vi "Create VI Snippets.vi"(6 "Skip":cluster{"Functions":i32[], "Controls":i32[]}={"Functions"=[2371, 2060], "Controls"=[3503, 21820]}, 8 "error in (no error)":errorcluster, 9 "Scripting Ring":refnum<vi>, 10 "Type":enum8{"Functions", "Controls"}(ring), 11 "OutputDir":path) -> (0 "error out":errorcluster, 3 "IDs":i32[](array[numeric]))   [LabVIEW 2018, in "Export-Built-ins.lvlib"]
uses:
  Export-Built-ins.lvlib
  <vilib>/Utility/miscctls.llb/LVPointTypeDef.ctl
panel:
  out "Name":string
  out "Current":i32
  out "Last Snippet (.png)":path
  out "Image":picture
  out "Info":string
  out "Last":i32
  out "Remaining":i32
  out "LabVIEW 2018 Scripting Ring":i32(ring)=2125 items=[".NET Container"=2125, ".NET Refnum"=3441, "2D Picture"=3508, "3D Picture"=23776, "Absolute Value"=1054, "Access Rights"=1412, "ActiveX Container"=2072, "Add"=1050, "Add (with error terminals)"=3915, "Add Array Elements"=1903, "Agitator"=3831, "AllSpoll"=1960, "Always Copy"=2400, "And"=1061, "And Array Elements"=1911, "Append True/False String"=1511, "Application Refnum"=3412, "Array (block diagram constant)"=2070, "Array (classic)"=3300, "Array (modern)"=21608, "Array Interface Control"=23777, "Array Max & Min"=1907, "Array of Strings to Path"=1422, "Array Size"=1809, "Array Subset"=2044, "Array To Cluster"=1168, "Array To Spreadsheet String"=1540, "ArrayMemInfo"=2412, "Assert Structural Type Match"=2416, "Atmospheric Tank (classic)"=3070, "Atmospheric Tank (modern)"=21751, "Automation Close"=8001, "Automation Open"=8000, "Automation Refnum"=3410, "Avogadro Constant (1/mol)"=23520, "Base 10 Logarithm Of e"=23512, "Bin #1"=3073, "Bin #2"=21755, "Bitpack to Array"=3135, "Bluetooth Close Connection"=9148, "Bluetooth Create Listener"=9151, "Bluetooth Discover"=9152, "Bluetooth Network Connection Refnum"=3468, "Bluetooth Open Connection"=9153, "Bluetooth Read"=9149, "Bluetooth Wait On Listener"=9147, "Bluetooth Write"=9150, "Boolean Array To Number"=1815, "Boolean To (0,1)"=1167, "Build Array"=2041, "Build Cluster Array"=2047, "Build Matrix"=8500, "Build Path"=1419, "Build Waveform"=2066, "Bundle"=2049, "Bundle By Name"=2057, "Byte Array To String"=1609, "Byte Stream File Refnum"=3408, "Call By Reference"=3901, "Call Chain"=1999, "Call Library Function Node"=2062, "Call Parent Method"=2354, "CAN Channel (block diagram constant)"=2124, "CAN Channel (classic)"=3340, "CAN Channel (modern)"=21817, "CAN Channel (system)"=21966, "CAN Interface (block diagram constant)"=2123, "CAN Interface (classic)"=3339, "CAN Interface (modern)"=21815, "CAN Interface (system)"=21964, "CAN Task (block diagram constant)"=3471, "CAN Task (classic)"=3470, "CAN Task (modern)"=21789, "CAN Task (system)"=21963, "Cancel Button (modern)"=21739, "Cancel Button (system)"=3131, "Cancel Notification"=9107, "Carriage Return Constant"=23500, "Case Structure"=2001, "Cast Unit Bases"=1079, "Check Valve"=3833, "Checkbox (classic)"=3117, "CheckBox (modern)"=21924, "Checkbox (system)"=3132, "Class Specifier Constant"=2094, "Classic Color Box"=3013, "Classic Color Ramp"=3022, "Classic Horizontal Slide Switch"=3114, "Classic Vertical Slide"=3004, "Clear Fixed-Point Overflow Status"=5562, "Close File"=8052, "Close File (deprecated)"=1405, "Close Python Session"=24207, "Close Reference"=8011, "Close Variable Connection"=23783, "Closure Structure"=2372, "Cluster (classic)"=3400, "Cluster (modern)"=21607, "Cluster Constant"=2071, "Cluster To Array"=1169, "Code Interface Node"=2050, "Coerce To Type"=2402, "Color Box Constant"=2120, "Color Box Thin Border"=2905, "Colored Rectangle (broken?)"=3625, "Combo Box (classic)"=3304, "Combo Box (modern)"=21604, "Combo Box (system)"=21917, "Combo Box Constant"=2088, "Complex Conjugate"=1048, "Complex To Polar"=1045, "Complex To Re/Im"=1044, "Compound Arithmetic"=2200, "Compressor"=3832, "Concatenate Strings"=2040, "Conditional Disable Structure"=2064, "Constructor Node"=3904, "Control & Simulation Loop"=2099, "Control Help Window"=1353, "Control Online Help"=1355, "Control Refnum"=3419, "Convert Unit"=2059, "Conveyer"=3827, "Copy"=8053, "Copy (deprecated)"=1416, "Cosecant"=1204, "Cosine"=1201, "Cotangent"=1205, "CPU Information"=24130, "Create Folder"=8055, "Create Network Stream Endpoint"=23793, "Create Network Stream Reader Endpoint"=23811, "Create Network Stream Writer Endpoint"=23810, "Create Stream"=23796, "Create Unique Network Stream Endpoint"=23795, "Create Unique Network Stream Reader Endpoint"=23807, "Create Unique Network Stream Writer Endpoint"=23806, "Create User Event"=2073, "Current Processor ID"=24131, "Current VI's Menubar"=9000, "Current VI's Path"=1426, "DAQmx Analog Trigger Source (block diagram constant)"=2119, "DAQmx Analog Trigger Source (classic)"=3336, "DAQmx Analog Trigger Source (modern)"=21774, "DAQmx Analog Trigger Source (system)"=21951, "DAQmx Device Name (block diagram constant)"=2093, "DAQmx Device Name (classic)"=3318, "DAQmx Device Name (modern)"=21773, "DAQmx Device Name (system)"=21950, "DAQmx Global Channel (block diagram constant)"=3430, "DAQmx Global Channel (classic)"=3443, "DAQmx Global Channel (modern)"=21770, "DAQmx Global Channel (system)"=21957, "DAQmx Physical Channel (block diagram constant)"=2118, "DAQmx Physical Channel (classic)"=3335, "DAQmx Physical Channel (modern)"=21777, "DAQmx Physical Channel (system)"=21954, "DAQmx Scale Name (block diagram constant)"=2116, "DAQmx Scale Name (classic)"=3317, "DAQmx Scale Name (modern)"=21775, "DAQmx Scale Name (system)"=21952, "DAQmx Switch (block diagram constant)"=2121, "DAQmx Switch (classic)"=3337, "DAQmx Switch (modern)"=21776, "DAQmx Switch (system)"=21953, "DAQmx Task Name (block diagram constant)"=3434, "DAQmx Task Name (classic)"=3442, "DAQmx Task Name (modern)"=21778, "DAQmx Task Name (system)"=21959, "DAQmx Terminal (block diagram constant)"=2117, "DAQmx Terminal (classic)"=3319, "DAQmx Terminal (modern)"=21781, "DAQmx Terminal (system)"=21955, "Data Cache Size"=24132, "Data Log File Refnum"=3402, "Data Value Reference"=3476, "Data Value Reference Constant"=24134, "DataSocket Close"=1085, "DataSocket Open"=1084, "DataSocket Read"=1086, "DataSocket Refnum"=3417, "DataSocket Write"=1087, "Date/Time To Seconds"=1308, "Decimal Digit?"=1119, "Decimal String To Number"=1184, "Decimate 1D Array"=2046, "DecomposeLockDataValRef"=2406, "DecomposeVariant"=2404, "Decrement"=1058, "Default Directory"=1427, "Delete"=8056, "Delete (deprecated)"=1417, "Delete Data Value Reference"=2409, "Delete From Array"=3912, "Delete Menu Items"=9004, "Delete Variant Attribute"=8206, "Delete Waveform Attribute"=8209, "Deny Access"=8057, "Dequeue Element"=9113, "Destroy Stream Endpoint"=23794, "Destroy User Event"=2075, "DevClear"=1961, "DevClearList"=1962, "Device Control/Status"=1433, "Device Refnum"=3405, "Diagram Disable Structure"=2054, "Dial (classic)"=3050, "Dial (modern)"=21732, "Digital Data (classic)"=3210, "Digital Data (modern)"=21216, "Digital Waveform Graph (classic)"=3511, "Digital Waveform Graph (modern)"=21718, "Direct Variable Read"=23785, "Direct Variable Write"=23788, "Divide"=1053, "Divide (with error terminals)"=3918, "Dlg Horiz Scrollbar"=21905, "Dlg Mac Group Box"=32514, "Dlg Numeric #1"=2100, "Dlg Numeric #2"=3006, "Dlg String"=2110, "Dlg Vert Scrollbar"=21906, "Down Arrow"=3824, "Down Bow Valve (flat)"=3707, "Down Bow Valve (outline)"=3807, "Down Bow Valve (shaded)"=21767, "Down Rect Valve (flat)"=3706, "Down Rect Valve (outline)"=3806, "Down Rect Valve (shaded)"=21766, "Down Tee (flat)"=3818, "Down Tee (shaded)"=3718, "Dynamic FPGA Interface Cast"=5690, "Eased Corner Rectangle"=32513, "Elementary Charge (C)"=23517, "Empty Array?"=23063, "Empty Path Constant"=23523, "Empty String Constant"=23503, "Empty String/Path?"=1112, "Enable Menu Tracking"=9002, "EnableLocal"=1963, "EnableRemote"=1964, "End of Line Constant"=23525, "Enqueue Element"=9111, "Enqueue Element At Opposite End"=9129, "Enum (classic)"=3023, "Enum (modern)"=21605, "Enum (system)"=3062, "Enum Constant"=2090, "EOF"=1410, "Equal To 0?"=1113, "Equal?"=1102, "Error Ring Constant"=2039, "Event Callback Refnum"=3435, "Event Data Node"=2102, "Event Structure"=2052, "Exchanger"=3828, "Exclusive Or"=1063, "Exponential"=1211, "Exponential (Arg) -1"=1222, "Expression Node"=2201, "False Constant"=2006, "Feedback Node"=2353, "FieldPoint IO Point (block diagram constant)"=3440, "FieldPoint IO Point (classic)"=3439, "FieldPoint IO Point (modern)"=21784, "FIFO Refnum"=3474, "File Dialog"=8058, "File Dialog (deprecated)"=8081, "File Path Control (classic)"=3203, "File Path Control (modern)"=21730, "File Path Control (system)"=21922, "File Path Indicator (classic)"=3204, "File Path Indicator (modern)"=21731, "File/Directory Info"=8082, "File/Directory Info (deprecated)"=1413, "FindLstn"=1965, "FindRQS"=1966, "First Call?"=1083, "Fixed-Point Overflow?"=5565, "Fixed-Point to Integer Cast"=5566, "Flat Box"=3602, "Flat Circle"=3605, "Flat Down Triangle"=3623, "Flat Frame"=3608, "Flat Left Triangle"=3620, "Flat Right Triangle"=3621, "Flat Round Button"=3102, "Flat Rounded Box"=3611, "Flat Sequence Structure"=2069, "Flat Square Button"=3103, "Flat Up Triangle"=3622, "Flatten To JSON"=24201, "Flatten To String"=1164, "Flatten To XML"=8400, "Flattened String To Variant"=8202, "Floating Point Equal?"=23064, "Flush Event Queue"=2135, "Flush File"=8059, "Flush File (deprecated)"=1406, "Flush Queue"=9114, "Flush Stream"=23808, "For Loop"=2002, "Fork"=2194, "Format Date/Time String"=8100, "Format Into File"=2083, "Format Into String"=2081, "Format Value"=1512, "Formula Node"=2004, "FPGA Refnum to Session"=2322, "Fract/Exp String To Number"=1187, "Framed Color Box (classic)"=3008, "Framed Color Box (modern)"=21019, "Free Label"=2321, "Furnace"=3829, "Gauge (classic)"=3040, "Gauge (modern)"=21009, "Gauge for Simon"=32600, "Generate Front Panel Activity"=1329, "Generate Occurrence"=1700, "Generate User Event"=2074, "Generate User-Defined Trace Event"=2250, "Get Control Values by Index"=24204, "Get Datalog Position"=8061, "Get Date/Time In Seconds"=1303, "Get Date/Time String"=1600, "Get Drag Drop Data"=9154, "Get File Position"=8062, "Get File Size"=8063, "Get Fixed-Point Components"=11163, "Get Help Window Status"=1354, "Get Matrix Diagonal"=8501, "Get Matrix Elements"=8502, "Get Menu Item Info"=9005, "Get Menu Selection"=9001, "Get Menu Short Cut Info"=9007, "Get Notifier Status"=9103, "Get Number of Records"=8064, "Get Permissions"=8065, "Get Queue Status"=9110, "Get Submatrix"=8503, "Get Type and Creator"=8066, "Get Variant Attribute"=8205, "Get Volume Info"=8067, "Get Waveform Attribute"=8208, "Get Waveform Components"=2067, "Global Variable"=2060, "GPIB Clear"=1954, "GPIB Initialization"=1957, "GPIB Misc"=1956, "GPIB Read"=1951, "GPIB Serial Poll"=1955, "GPIB Status"=1959, "GPIB Trigger"=1953, "GPIB Wait"=1958, "GPIB Write"=1950, "Gravitational Constant (N m2/kg2)"=23519, "Greater Or Equal To 0?"=1114, "Greater Or Equal?"=1103, "Greater Than 0?"=1117, "Greater?"=1110, "Handle Peek"=1604, "Handle Poke"=1605, "Hex Digit?"=1123, "Hexadecimal String To Number"=1185, "Hopper #1"=21754, "Hopper #2"=3072, "Horiz Line"=3821, "Horiz Pipe (flat)"=3810, "Horiz Pipe (shaded)"=3710, "Horizontal Button Box"=3636, "Horizontal Fill Slide (classic)"=3012, "Horizontal Fill Slide (modern)"=21100, "Horizontal Gradient Oval"=32502, "Horizontal Gradient Rectangle"=32504, "Horizontal Gradient Rounded Rectangle"=32507, "Horizontal Graduated Bar"=21106, "Horizontal Pointer Slide (classic)"=3011, "Horizontal Pointer Slide (modern)"=21101, "Horizontal Pointer Slide (system)"=21902, "Horizontal Progress Bar (modern)"=21102, "Horizontal Progress Bar (system)"=21910, "Horizontal Scrollbar"=21110, "Horizontal Slide (classic)"=3010, "Horizontal Slide (system)"=21904, "Horizontal Smooth Box"=3633, "Horizontal Splitter Bar"=21861, "Horizontal Splitter Bar (Classic)"=21863, "Horizontal Splitter Bar (System)"=21865, "Horizontal Switch"=3108, "Horizontal Tank"=3071, "Horizontal Toggle Switch (classic)"=3110, "Horizontal Toggle Switch (modern)"=21700, "Hyperbolic Cosecant"=23053, "Hyperbolic Cosine"=1215, "Hyperbolic Cotangent"=23055, "Hyperbolic Secant"=23054, "Hyperbolic Sine"=1214, "Hyperbolic Tangent"=1216, "IMAQ Session"=3415, "Implies"=1080, "In Place Element Structure"=2360, "In Range and Coerce"=1127, "Include Fixed-Point Overflow Status"=5564, "Increment"=1057, "Index & Bundle Cluster Array"=2056, "Index Array"=2042, "Index String Array"=1531, "Initialize Array"=2053, "Inline C Node"=2104, "Insert Into Array"=3911, "Insert Menu Items"=9003, "Integer to Fixed-Point Cast"=5567, "Intensity Chart (classic)"=3509, "Intensity Chart (modern)"=21719, "Intensity Graph (classic)"=3510, "Intensity Graph (modern)"=21720, "Interleave 1D Arrays"=2045, "Interpolate 1D Array"=1905, "Inverse Cosecant"=23050, "Inverse Cosine"=1207, "Inverse Cotangent"=23052, "Inverse Hyperbolic Cosecant"=23056, "Inverse Hyperbolic Cosine"=1218, "Inverse Hyperbolic Cotangent"=23058, "Inverse Hyperbolic Secant"=23057, "Inverse Hyperbolic Sine"=1217, "Inverse Hyperbolic Tangent"=1219, "Inverse Secant"=23051, "Inverse Sine"=1206, "Inverse Tangent"=1208, "Inverse Tangent (2 Input)"=1228, "Invoke Node"=3900, "IP To String"=1710, "IrDA Close Connection"=9144, "IrDA Create Listener"=9140, "IrDA Discover"=9141, "IrDA Network Connection Refnum"=3450, "IrDA Open Connection"=9142, "IrDA Read"=9145, "IrDA Wait On Listener"=9143, "IrDA Write"=9146, "IVI Delete Session"=8103, "IVI Logical Name (block diagram constant)"=3420, "IVI Logical Name (classic)"=3414, "IVI Logical Name (modern)"=21736, "IVI New Session"=8102, "Join"=2195, "Join Numbers"=1171, "Junction"=2197, "Knob (classic)"=3005, "Knob (modern)"=21000, "Label (modern)"=21960, "Label (system)"=21961, "Labeled Oblong Button"=3125, "Labeled Rectangular Button"=3124, "Labeled Round Button"=3122, "Labeled Square Button"=3123, "LabVIEW Object"=3457, "Leak Variant Value Reference"=2410, "LED Button"=3116, "Left Arrow"=3826, "Left Bow Valve (flat)"=3701, "Left Bow Valve (outline)"=3801, "Left Bow Valve (shaded)"=21761, "Left Down Elbow (flat)"=3811, "Left Down Elbow (shaded)"=3711, "Left Pump (flat)"=3813, "Left Pump (shaded)"=3713, "Left Rect Valve (flat)"=3700, "Left Rect Valve (outline)"=3800, "Left Rect Valve (shaded)"=21760, "Left Tee (flat)"=3809, "Left Tee (shaded)"=3709, "Left Up Elbow (flat)"=3808, "Left Up Elbow (shaded)"=3708, "Less Or Equal To 0?"=1115, "Less Or Equal?"=1104, "Less Than 0?"=1118, "Less?"=1111, "Lexical Class"=1126, "Line (chiseled, system)"=3632, "Line (chiseled, thick)"=3630, "Line (chiseled, thin)"=3627, "Line (thick)"=3629, "Line (thin)"=3626, "Line Feed Constant"=23501, "Line with Arrow (thick)"=3631, "Line with Arrow (thin)"=3628, "List Directory"=1418, "List Folder"=8083, "Listbox (classic)"=21806, "Listbox (modern)"=21792, "Listbox (system)"=21805, "Listbox Symbol Ring Constant"=2038, "Local Variable"=2061, "Lock Range"=1411, "Logarithm Base 10"=1210, "Logarithm Base 2"=1225, "Logarithm Base X"=1224, "Logical Shift"=1081, "Lookup Channel Probe"=9155, "Lossy Enqueue Element"=9130, "Lowered Box (thick)"=3635, "Lowered Rounded Box"=3638, "Machine Epsilon"=23528, "MakeAddr"=1967, "Mantissa & Exponent"=1150, "Match First String"=1532, "Match Pattern"=1535, "Match True/False String"=1533, "MathScript Call By Reference"=3906, "MathScript Node"=2357, "MATLAB script"=9020, "Matrix Size"=8507, "Max & Min"=1108, "Menu Refnum"=3413, "Menu Ring (classic)"=3018, "Menu Ring (modern)"=21600, "Menu-Popup Ring"=3017, "Merge Errors"=2147, "Merge Signals"=2350, "Meter (classic)"=3030, "Meter (modern)"=21008, "Mixed Checkbox (system)"=21333, "Mixed Signal Graph"=21721, "Molar Gas Constant (J/(mol K))"=23522, "Motion Resource (block diagram constant)"=3449, "Motion Resource (classic)"=3448, "Motion Resource (modern)"=21787, "Motor (flat)"=3820, "Motor (shaded)"=3720, "Move"=8068, "Move (deprecated)"=1415, "Multi-Segment Pipe"=23780, "Multicolumn Listbox (classic)"=21799, "Multicolumn Listbox (modern)"=21791, "Multicolumn Listbox (system)"=21798, "Multiply"=1052, "Multiply (with error terminals)"=3917, "Multiply Array Elements"=1904, "Multirate Structure"=2199, "Natural Logarithm"=1209, "Natural Logarithm (Arg +1)"=1221, "Natural Logarithm Base"=23510, "Natural Logarithm Of 10"=23513, "Natural Logarithm Of 2"=23514, "Natural Logarithm Of Pi"=23508, "Negate"=1069, "Negative Infinity"=23509, "New Data Value Reference"=2408, "New Directory"=1402, "New File"=1404, "New VI"=8014, "New VI Object"=8015, "Not"=1064, "Not A Number/Path/Refnum?"=1128, "Not A Path Constant"=23524, "Not a Refnum Constant"=23526, "Not a Shared Variable"=23527, "Not And"=1071, "Not Equal To 0?"=1116, "Not Equal?"=1105, "Not Exclusive Or"=1073, "Not Or"=1072, "Notifier Refnum"=3423, "Number of Cache Levels"=24133, "Number To Boolean Array"=1814, "Number To Decimal String"=1180, "Number To Engineering String"=1183, "Number To Exponential String"=1505, "Number To Fractional String"=1506, "Number To Hexadecimal String"=1181, "Number To Octal String"=1182, "Numeric Constant"=2005, "Numeric Control (classic)"=3000, "Numeric Control (modern)"=21003, "Numeric Control (system)"=21919, "Numeric Indicator (classic)"=3001, "Numeric Indicator (modern)"=21004, "Obtain Notifier"=9101, "Obtain Queue"=9108, "Occurrence Refnum"=3406, "Octal Digit?"=1129, "Octal String To Number"=1186, "OK Button (modern)"=21738, "OK Button (system)"=3130, "Old VISA Open"=1921, "OLE Variant"=3150, "One Button Dialog"=1340, "Open and Verify Variable Connection"=23790, "Open Application Reference"=8012, "Open Device"=1430, "Open Dynamic Bitfile Reference"=5691, "Open File"=1403, "Open Python Session"=24206, "Open Tank (flat classic)"=21752, "Open Tank (shaded classic)"=3074, "Open Variable Connection"=23779, "Open Variable Connection in Background"=23791, "Open VI Object Reference"=8013, "Open VI Reference"=8010, "Open/Create/Replace Datalog"=8054, "Open/Create/Replace File"=8050, "Or"=1062, "Or Array Elements"=1910, "Oval with Shadow"=32509, "Package Matrix"=23001, "PassControl"=1968, "Path Constant"=2009, "Path to Array of Strings"=1423, "Path To String"=1077, "Path Type"=1421, "Pi"=23504, "Pi Divided By 2"=23506, "Pi Multiplied By 2"=23505, "Pick Line"=1510, "Pict Ring (classic)"=3015, "Pict Ring (modern)"=21602, "Pict Ring (system)"=21925, "PixMap"=3505, "PixMap (warning: dangerous)"=3507, "Planck's Constant (J/Hz)"=23516, "Platform Flat Square Button"=3134, "Plug-In Control"=21820, "Polar To Complex"=1047, "Polar To Re/Im"=23061, "Positive Infinity"=23515, "Power Of 10"=1212, "Power Of 2"=1223, "Power Of X"=1213, "PPoll"=1969, "PPollConfig"=1970, "PPollUnconfig"=1971, "Preallocated Read from Binary File"=24135, "Preserve Run-Time Class"=8018, "Pressure Tank (flat)"=3075, "Pressure Tank (shaded)"=21753, "Preview Queue Element"=9112, "Printable?"=1124, "Property Node"=1920, "Pulldown Menu Ring"=3061, "Push Button"=21001, "Python Node"=24205, "Python Session Refnum"=3486, "Queue Refnum"=3424, "Quit LabVIEW"=1352, "Quotient & Remainder"=1056, "Race Structure"=2371, "Radio Button (system)"=3133, "Radio Buttons (classic)"=22003, "Radio Buttons (modern)"=22001, "Radio Buttons (system)"=22002, "Raised Box (classic)"=3600, "Raised Box (modern)"=3637, "Raised Circle"=3603, "Raised Down Triangle"=3615, "Raised Frame"=3606, "Raised Left Triangle"=3612, "Raised Right Triangle"=3613, "Raised Rounded Box"=3609, "Raised Up Triangle"=3614, "Random Number (0-1)"=1070, "RcvRespMsg"=1972, "Re/Im To Complex"=1046, "Re/Im To Polar"=23060, "Read Datalog"=8069, "Read Device"=1432, "Read File"=1407, "Read from Binary File"=8051, "Read from Text File"=8070, "Read Multiple Elements from Stream"=23803, "Read Single Element from Stream"=23797, "Read Variable"=23781, "Read Variable with Timeout"=23786, "ReadStatus"=1973, "Receive"=1974, "ReceiveSetup"=1975, "Recessed Box"=3601, "Recessed Circle"=3604, "Recessed Down Triangle"=3619, "Recessed Frame (modern)"=3607, "Recessed Frame (system)"=3624, "Recessed Left Triangle"=3616, "Recessed Menu Ring"=3019, "Recessed Right Triangle"=3617, "Recessed Rounded Box"=3610, "Recessed Up Triangle"=3618, "Reciprocal"=1059, "Reciprocal Of e"=23511, "Reciprocal Of Pi"=23507, "RecomposeArray"=2403, "RecomposeUnlockDataValRef (warning: dangerous)"=2407, "RecomposeVariant (warning: dangerous)"=2405, "Rectangular Stop Button"=3128, "Refnum to Path"=1424, "Refnum to Session"=2306, "Region"=2196, "Register Event Callback"=2078, "Register For Events"=2065, "Register Session"=2319, "Release Notifier"=9102, "Release Queue"=9109, "Remove Fixed-Point Overflow Status"=5563, "Replace Array Subset"=3910, "Replace Substring"=3913, "Request Deallocation"=1610, "ResetSys"=1976, "Reshape Array"=2055, "Resize Matrix"=8508, "Resource Index"=1088, "Reverse 1D Array"=1900, "Reverse String"=1537, "Right Arrow"=3825, "Right Bow Valve (flat)"=3705, "Right Bow Valve (outline)"=3805, "Right Bow Valve (shaded)"=21765, "Right Down Elbow (flat)"=3817, "Right Down Elbow (shaded)"=3717, "Right Pump (flat)"=3819, "Right Pump (shaded)"=3719, "Right Rect Valve (flat)"=3704, "Right Rect Valve (outline)"=3804, "Right Rect Valve (shaded)"=21764, "Right Tee (flat)"=3815, "Right Tee (shaded)"=3715, "Right Up Elbow (flat)"=3814, "Right Up Elbow (shaded)"=3714, "Rocker"=21002, "Rotary Feeder"=3830, "Rotate"=1082, "Rotate 1D Array"=1906, "Rotate Left With Carry"=1606, "Rotate Right With Carry"=1607, "Rotate String"=1536, "Round Button"=3100, "Round LED (classic)"=3120, "Round LED (modern)"=21012, "Round Light"=3104, "Round Push Button"=3118, "Round Push Button (profile)"=3112, "Round Radio Button"=3106, "Round Stop Button"=3127, "Round To Nearest"=1055, "Round Toward +Infinity"=1076, "Round Toward -Infinity"=1075, "Rounded Rectangle with Shadow"=32508, "RT FIFO Create"=24000, "RT FIFO Delete"=24003, "RT FIFO Read"=24001, "RT FIFO Write"=24002, "Rydberg Constant (1/m)"=23521, "Scale By Power Of 2"=1074, "Scan From File"=2082, "Scan From String"=2080, "Scan String For Tokens"=8101, "Scan Value"=1534, "Scanned Variable Read"=23784, "Scanned Variable Write"=23787, "Search 1D Array"=1901, "Search and Replace String"=3914, "Search Variable Container"=23802, "Search/Split String"=1538, "Secant"=1203, "Seconds To Date/Time"=1309, "Seek"=1409, "Select"=1516, "Send"=1977, "Send Notification"=9104, "SendCmds"=1978, "SendDataBytes"=1979, "SendIFC"=1980, "SendList"=1981, "SendLLO"=1982, "SendSetup"=1983, "Session to Refnum"=2307, "Set Control Values by Index"=24203, "Set Datalog Position"=8072, "Set File Position"=8073, "Set File Size"=8074, "Set Matrix Diagonal"=8504, "Set Matrix Elements"=8505, "Set Menu Item Info"=9006, "Set Number of Records"=8075, "Set Occurrence"=1702, "Set Permissions"=8076, "Set Submatrix"=8506, "Set Type and Creator"=8077, "Set Variant Attribute"=8204, "Set Waveform Attribute"=8207, "SetRWLS"=1984, "SetTimeOut"=1985, "Shared Variable"=23778, "Shared Variable Constant"=3473, "Shared Variable Control (classic)"=3472, "Shared Variable Control (modern)"=21814, "Shared Variable to String"=1831, "Sign"=1049, "Simple Horizontal Slide"=3003, "Simple Numeric"=2900, "Simple String"=2115, "Simple Vertical Slide"=3002, "Sinc"=1227, "Sine"=1200, "Sine & Cosine"=1220, "Size Handle"=1603, "Slide Switch"=21011, "Smoothed Oval"=32500, "Smoothed Rounded Rectangle"=32505, "Sort 1D Array"=1120, "Sort Array of String"=23065, "Speed Of Light In Vacuum (m/sec)"=23518, "Spin Control (system)"=21900, "Split 1D Array"=1908, "Split Button"=21020, "Split Number"=1170, "Split Signals"=2351, "Spreadsheet String To Array"=1539, "Square"=23059, "Square Button"=3101, "Square LED (classic)"=3121, "Square LED (modern)"=21013, "Square Light"=3105, "Square Push Button"=3119, "Square Push Button (profile)"=3113, "Square Radio Button"=3107, "Square Root"=1060, "Stacked Sequence Structure"=2000, "State"=2198, "State Diagram"=2051, "Static VI Reference"=2084, "Stop"=1350, "Stop Button"=21230, "String Constant"=2007, "String Control (classic)"=3200, "String Control (modern)"=21701, "String Control (system)"=21920, "String Indicator (classic)"=3201, "String Indicator (modern)"=21702, "String Length"=1502, "String Subset"=1503, "String To Byte Array"=1608, "String To IP"=1711, "String To Path"=1078, "String to Shared Variable"=1830, "Strip Path"=1420, "SubPanel"=21810, "SubPanel (Classic)"=21811, "SubPanel (System)"=21823, "Subtract"=1051, "Subtract (with error terminals)"=3916, "Swap Bytes"=1162, "Swap Values"=2401, "Swap Vector Element"=1912, "Swap Words"=1163, "Tab Constant"=23502, "Tab Control (classic)"=3330, "Tab Control (modern)"=3332, "Tab Control (NXG Style)"=32700, "Tab Control (system)"=3331, "Table (classic)"=21796, "Table (modern)"=21790, "Table (system)"=21797, "Tag Attribute Ring"=2063, "Tangent"=1202, "Tank (classic)"=3020, "Tank (modern)"=21006, "Target Structure"=2370, "TCP Close Connection"=1713, "TCP Create Listener"=1717, "TCP Flattened Read"=1718, "TCP Flattened Write"=1719, "TCP Flex Read"=1720, "TCP Flex Write"=1721, "TCP Network Connection Refnum"=3407, "TCP Open Connection"=1715, "TCP Read"=1716, "TCP Wait On Listener"=1712, "TCP Write"=1714, "TDMS Advanced Asynchronous Read (Data Ref)"=2151, "TDMS Advanced Asynchronous Write (Data Ref)"=2150, "TDMS Close"=24113, "TDMS Configure Asynchronous Reads (Data Ref)"=2153, "TDMS Configure Asynchronous Writes (Data Ref)"=2152, "TDMS Defragment"=24119, "TDMS Delete Data"=2159, "TDMS File"=3477, "TDMS Flush"=24117, "TDMS Get Asynchronous Read Status (Data Ref)"=2155, "TDMS Get Asynchronous Write Status (Data Ref)"=2154, "TDMS Get Properties"=24115, "TDMS In Memory Close"=2157, "TDMS In Memory Open"=2156, "TDMS In Memory Read Bytes"=2158, "TDMS List Contents"=24116, "TDMS Open"=24112, "TDMS Read"=24111, "TDMS Refnum To File ID"=24120, "TDMS Set Properties"=24114, "TDMS Write"=24110, "TDMS Write IP"=24118, "Temporary Directory"=1435, "TestSRQ"=1986, "TestSys"=1987, "Text & Pict Ring (classic)"=3016, "Text & Pict Ring (modern)"=21603, "Text Button"=21015, "Text Ring (block diagram constant)"=2008, "Text Ring (classic)"=3014, "Text Ring (modern)"=21601, "Text Ring (system)"=3060, "Text to UTF-8"=23066, "Thermometer (classic)"=3021, "Thermometer (modern)"=21007, "Threshold 1D Array"=1909, "Tick Count (ms)"=1300, "Time Stamp (block diagram constant)"=2068, "Time Stamp Control (classic)"=5555, "Time Stamp Control (modern)"=21913, "Time Stamp Control (system)"=21967, "Time Stamp Indicator (classic)"=5556, "Time Stamp Indicator (modern)"=21914, "Timed Loop"=5570, "Timed Sequence"=5573, "To Byte Integer"=1140, "To Double Precision Complex"=1152, "To Double Precision Float"=1147, "To Extended Precision Complex"=1154, "To Extended Precision Float"=1149, "To Fixed-Point"=5561, "To Long Integer"=1142, "To Lower Case"=1189, "To More Generic Class"=8017, "To More Specific Class"=8016, "To OLE Variant"=8002, "To Probe String"=2413, "To Quad Integer"=1155, "To Single Precision Complex"=1151, "To Single Precision Float"=1146, "To Time Stamp"=5560, "To Unsigned Byte Integer"=1143, "To Unsigned Long Integer"=1145, "To Unsigned Quad Integer"=1156, "To Unsigned Word Integer"=1144, "To Upper Case"=1188, "To Variant"=8201, "To Word Integer"=1141, "Traditional DAQ Channel (block diagram constant)"=2085, "Traditional DAQ Channel (classic)"=3320, "Traditional DAQ Channel (modern)"=21733, "Transpose 1D Array"=23068, "Transpose 2D Array"=1902, "Transpose Matrix"=8509, "Tree (classic)"=21819, "Tree (modern)"=21793, "Tree (system)"=21794, "Trigger"=1988, "TriggerList"=1989, "Two Button Dialog"=1341, "Type and Creator"=1434, "Type Cast"=1166, "Type Error"=2415, "Type Must Be Array"=2417, "Type Must Be Cluster"=2418, "Type Of"=2414, "Type Specialization Structure"=2373, "UDP Close"=1726, "UDP Multicast Open"=1727, "UDP Network Connection Refnum"=3418, "UDP Open"=1723, "UDP Read"=1724, "UDP Write"=1725, "Unbitpack from Array"=3136, "Unbundle"=2048, "Unbundle By Name"=2058, "Unflatten From JSON"=24202, "Unflatten From String"=1165, "Unflatten From XML"=8401, "Unleak Variant Value Reference"=2411, "Unpackage Matrix"=23000, "Unregister For Events"=2076, "Unregister Session"=2320, "Up Arrow"=3823, "Up Bow Valve (flat)"=3703, "Up Bow Valve (outline)"=3803, "Up Bow Valve (shaded)"=21763, "Up Rect Valve (flat)"=3702, "Up Rect Valve (outline)"=21762, "Up Rect Valve (shaded)"=3802, "Up Tee (flat)"=3812, "Up Tee (shaded)"=3712, "User Defined Refnum"=3428, "User Defined Refnum Tag (block diagram constant)"=3426, "User Defined Refnum Tag (classic)"=3429, "User Defined Refnum Tag (modern)"=21745, "User Defined Refnum Tag Flatten (classic)"=3454, "User Defined Refnum Tag Flatten (modern)"=21747, "User Defined Tag (block diagram constant)"=2114, "User Defined Tag (classic)"=3329, "User Defined Tag (modern)"=21749, "User Item"=3506, "UTF-8 to Text"=23067, "Variable Class Specifier Constant"=2106, "Variable Name Constant"=3478, "Variant"=3310, "Variant To Data"=8003, "Variant To Flattened String"=8203, "Vert Line"=3822, "Vert Pipe (flat)"=3816, "Vert Pipe (shaded)"=3716, "Vert Rocker"=21740, "Vertical Fill Slide (classic)"=3009, "Vertical Fill Slide (modern)"=21014, "Vertical Gradient Oval"=32501, "Vertical Gradient Rectangle"=32503, "Vertical Gradient Rounded Rectangle"=32506, "Vertical Graduated Bar"=21107, "Vertical Pointer Slide (classic)"=3007, "Vertical Pointer Slide (modern)"=21017, "Vertical Pointer Slide (system)"=21901, "Vertical Progress Bar (modern)"=21104, "Vertical Progress Bar (system)"=21909, "Vertical Scrollbar"=21111, "Vertical Slide (system)"=21903, "Vertical Slide Switch (classic)"=3115, "Vertical Slide Switch (modern)"=21741, "Vertical Smooth Box"=3634, "Vertical Splitter Bar"=21860, "Vertical Splitter Bar (Classic)"=21862, "Vertical Splitter Bar (System)"=21864, "Vertical Switch"=3109, "Vertical Toggle Switch (classic)"=3111, "Vertical Toggle Switch (modern)"=21005, "VI Library"=1425, "VI Refnum"=3422, "VI Server Reference"=2091, "VISA Assert Interrupt Signal"=2309, "VISA Assert Trigger"=1929, "VISA Assert Utility Signal"=2310, "VISA Clear"=1927, "VISA Close"=1922, "VISA Disable Event"=1940, "VISA Discard Events"=1941, "VISA Enable Event"=1942, "VISA Find Resource"=1923, "VISA Flush I/O Buffer"=2302, "VISA GPIB Command"=2315, "VISA GPIB Control ATN"=2316, "VISA GPIB Control REN"=2304, "VISA GPIB Pass Control"=2317, "VISA GPIB Send IFC"=2318, "VISA In 16"=1930, "VISA In 32"=1944, "VISA In 64"=2140, "VISA In 8"=1936, "VISA Lock"=1993, "VISA Map Address"=1932, "VISA Map Trigger"=2311, "VISA Memory Allocation"=1997, "VISA Memory Allocation Ex"=2146, "VISA Memory Free"=1998, "VISA Move"=2303, "VISA Move In 16"=1948, "VISA Move In 32"=1991, "VISA Move In 64"=2144, "VISA Move In 8"=1946, "VISA Move Out 16"=1949, "VISA Move Out 32"=1992, "VISA Move Out 64"=2145, "VISA Move Out 8"=1947, "VISA Open"=2308, "VISA Out 16"=1931, "VISA Out 32"=1945, "VISA Out 64"=2141, "VISA Out 8"=1937, "VISA Peek 16"=1934, "VISA Peek 32"=1995, "VISA Peek 64"=2142, "VISA Peek 8"=1938, "VISA Poke 16"=1935, "VISA Poke 32"=1996, "VISA Poke 64"=2143, "VISA Poke 8"=1939, "VISA Read"=1925, "VISA Read STB"=1928, "VISA Read To File"=2313, "VISA Refnum to Session"=2300, "VISA Resource Name"=3421, "VISA resource name (classic)"=3409, "VISA resource name (modern)"=21737, "VISA Set I/O Buffer Size"=2301, "VISA Status Description"=1924, "VISA Unlock"=1994, "VISA Unmap Address"=1933, "VISA Unmap Trigger"=2312, "VISA USB Control In"=2086, "VISA USB Control Out"=2087, "VISA VXI Cmd or Query"=2305, "VISA Wait on Event"=1943, "VISA Write"=1926, "VISA Write From File"=2314, "Volume Info"=1414, "Wait (ms)"=1302, "Wait For Activity"=1722, "Wait For Front Panel Activity"=1328, "Wait for GPIB RQS"=1952, "Wait on Notification"=9105, "Wait on Notification from Multiple"=9106, "Wait on Notification from Multiple with Notifier History"=9132, "Wait on Notification with Notifier History"=9131, "Wait on Occurrence"=1701, "Wait Until Next ms Multiple"=1327, "WaitSRQ"=1990, "Waveform Chart"=21010, "Waveform Chart (classic)"=3501, "Waveform Chart (modern)"=21717, "Waveform Graph (classic)"=3504, "Waveform Graph (modern)"=21703, "While Loop #1"=2003, "While Loop #2"=2352, "White Space?"=1125, "Write Datalog"=8079, "Write Device"=1431, "Write File"=1408, "Write Multiple Elements to Stream"=23804, "Write Single Element to Stream"=23798, "Write to Binary File"=8078, "Write to Text File"=8080, "Write Variable"=23782, "Write Variable with Timeout"=23789, "XY Graph (classic)"=3500, "XY Graph (modern)"=21716, "Y-th Root of X"=23062]
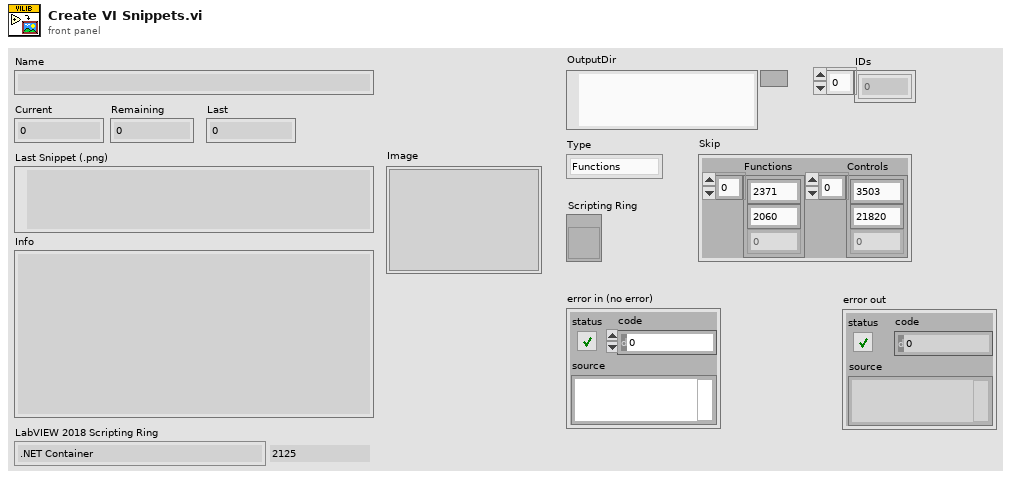
[diagram p1: front panel]
types:
  T1 = enum16{"open", "replace", "create", "open or create", "replace or create", "replace or create with confirmation"}
  T2 = typedef "LVStringsAndValuesArrayTypeDef_I32.ctl" = cluster{"String":string, "Value":i32}[]
  T3 = typedef "LVPointTypeDef.ctl" = cluster{"Horizontal":i16, "Vertical":i16}
  T4 = typedef "LVRectTypeDef.ctl" = cluster{"Left":i16, "Top":i16, "Right":i16, "Bottom":i16}
  T5 = typedef "imagedata.ctl" = cluster{"image type":i32, "image depth":i32, "image":u8[], "mask":u8[], "colors":u32[], "Rectangle":cluster{"left":i16, "top":i16, "right":i16, "bottom":i16}}
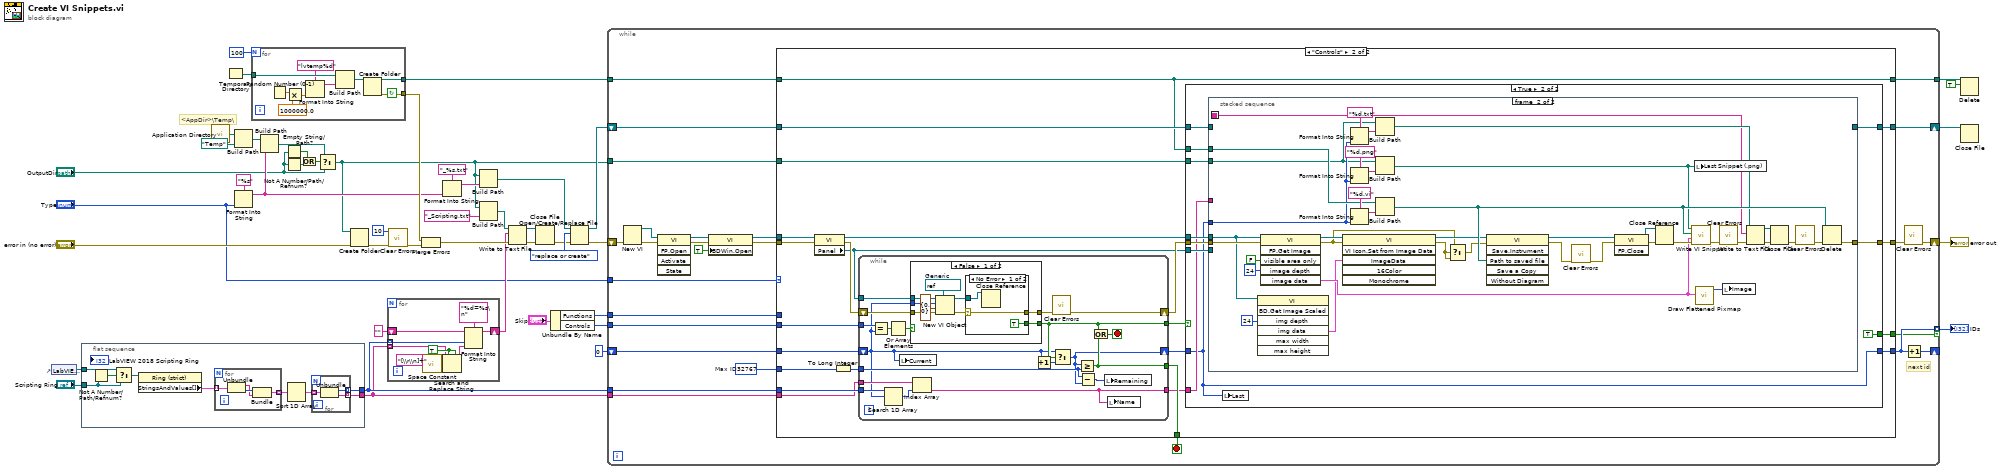
[diagram p0: block diagram]
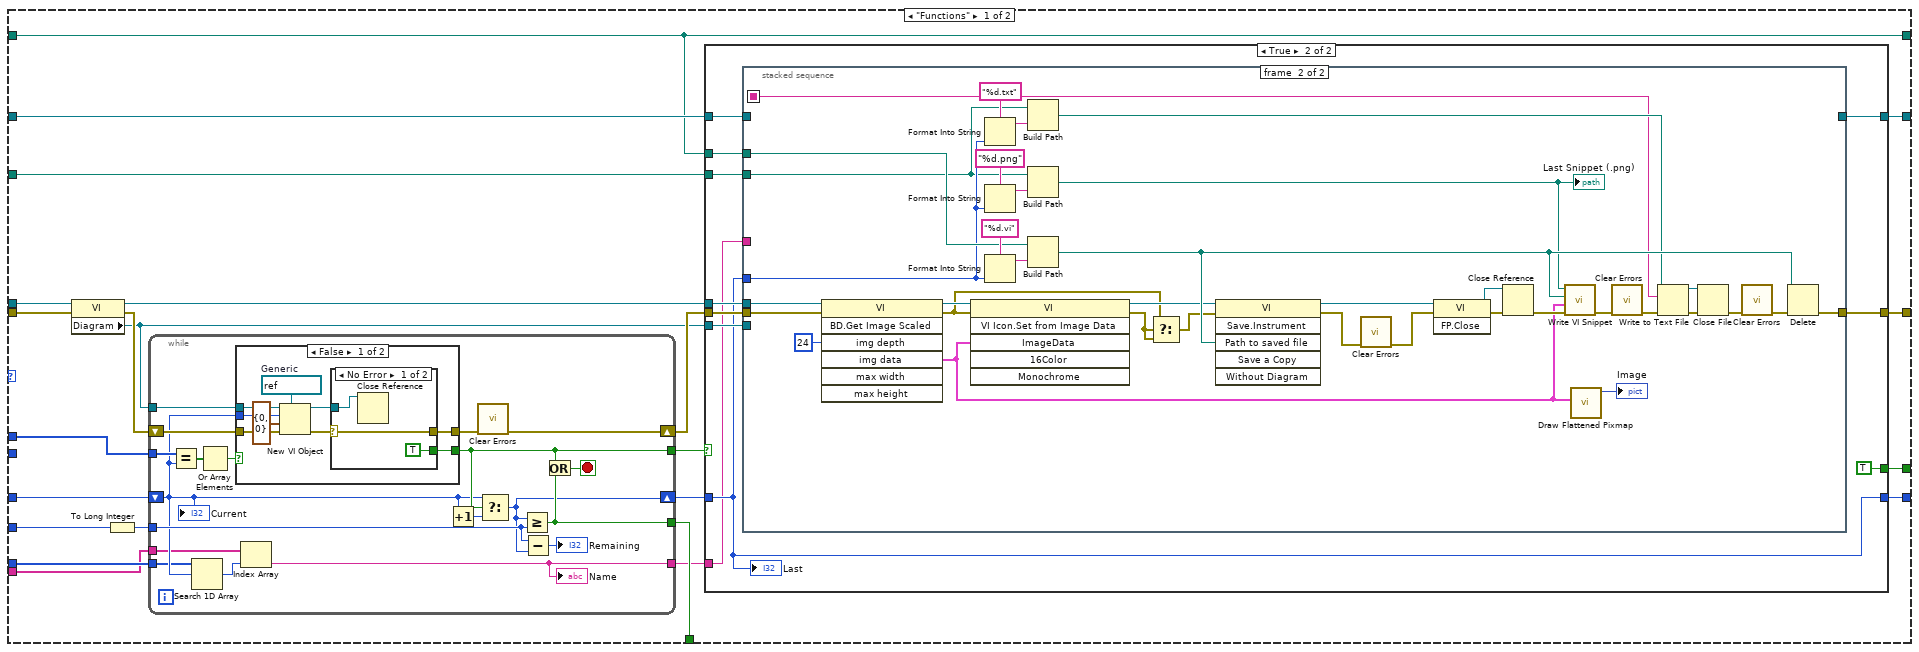
[diagram p2: hidden frame]
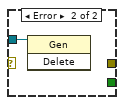
[diagram p3: hidden frame]
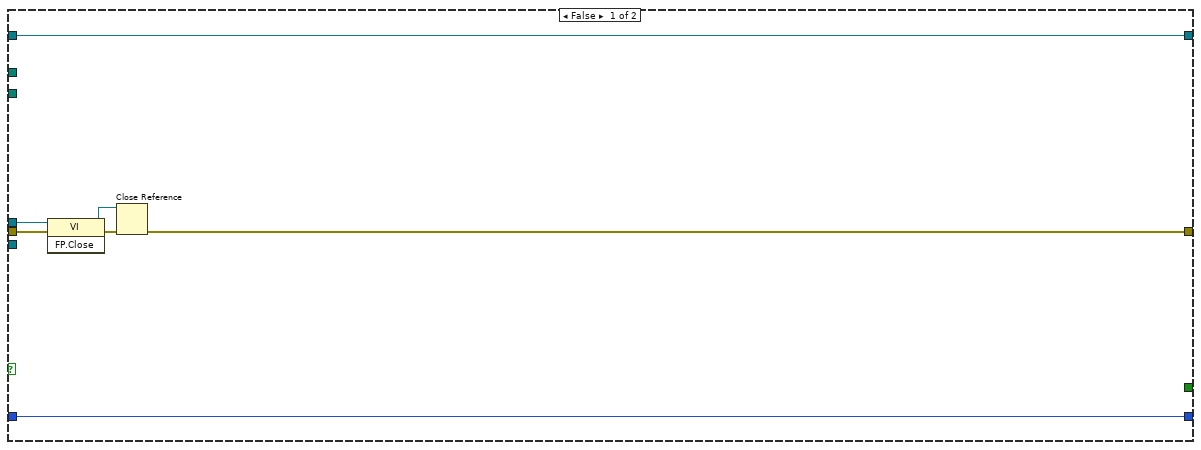
[diagram p5: hidden frame]
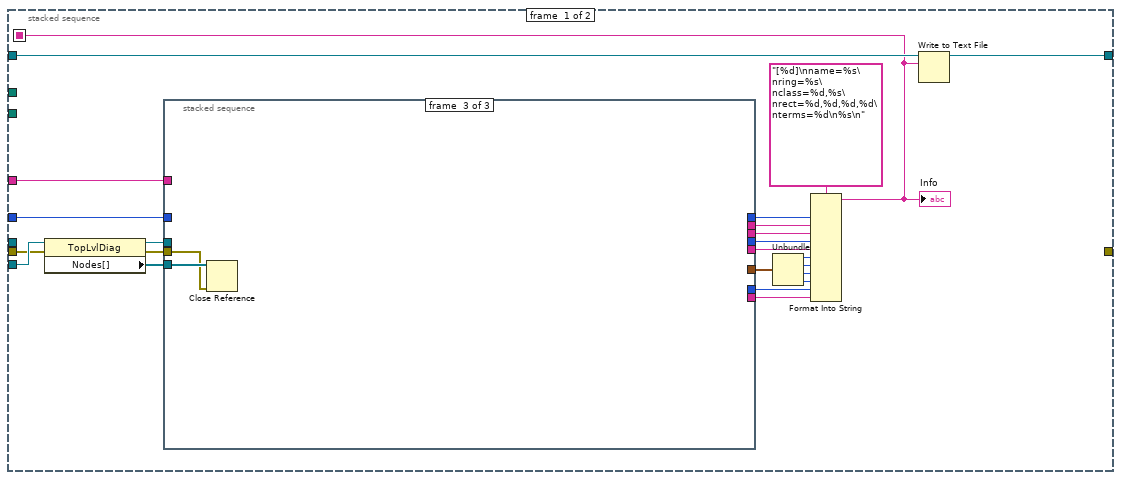
[diagram p6: hidden frame]
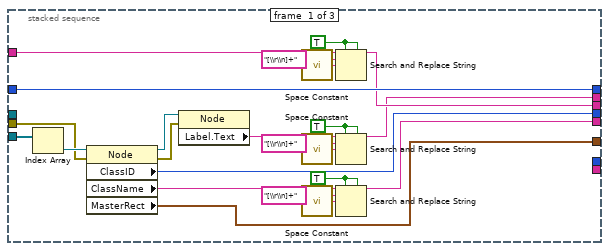
[diagram p7: hidden frame]
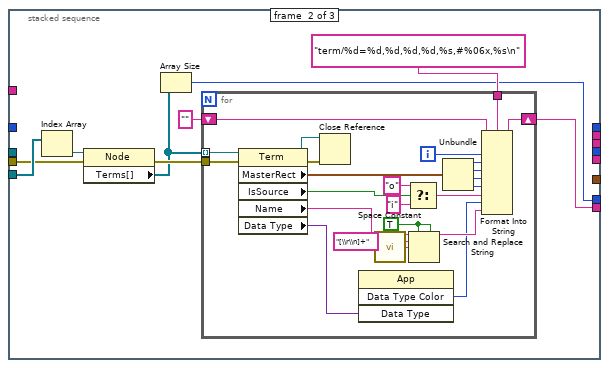
[diagram p8: hidden frame]
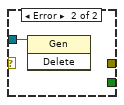
[diagram p9: hidden frame]
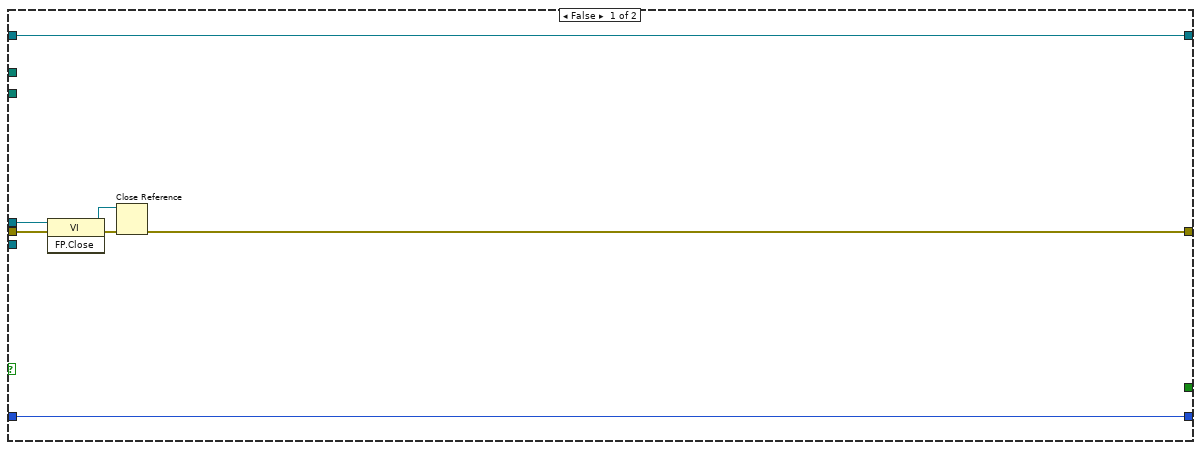
[diagram p11: hidden frame]
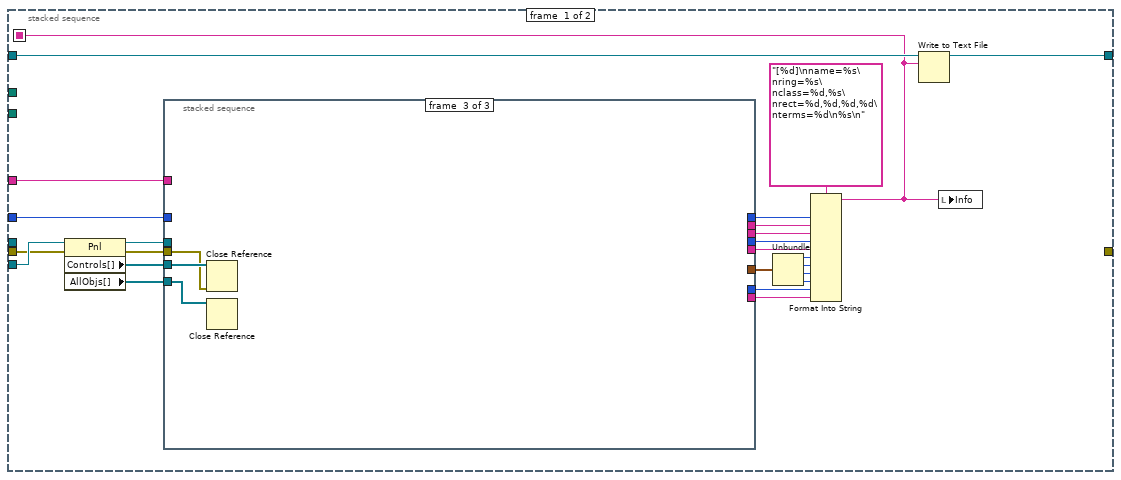
[diagram p12: hidden frame]
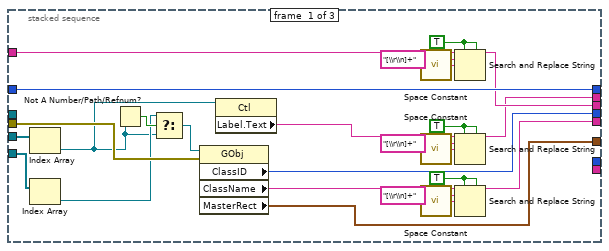
[diagram p13: hidden frame]
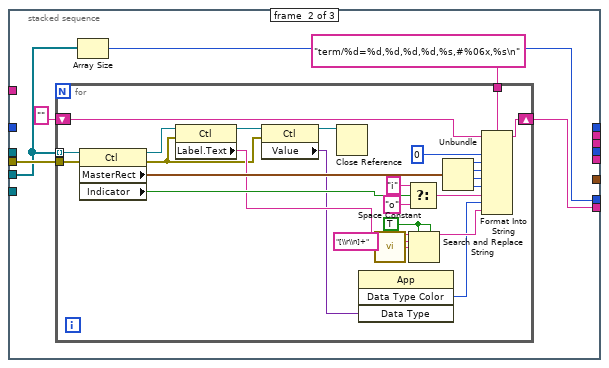
[diagram p14: hidden frame]
diagram:
  # "<AppDir>\\Temp\\"
  n1 = control-ref of="LabVIEW 2018 Scripting Ring"() -> (w7:refnum<vi>)
  n2 = flat-sequence {
    tunnel: [w53] -> w6
    tunnel: [w52] -> w5
    tunnel: "Scripting Ring" -> [w49]
    tunnel: w7 -> [w48]
    frame #0 {
      n3 = Not A Number/Path/Refnum?(number/path/refnum=w49) -> (NaN/Path/Refnum?=w51:bool)
      n4 = Select(t=w48, s=w51, f=w49) -> (s? t:f=w50:refnum<vi>)
      n5 = property on="Property Node" class="Ring (strict)"(reference=w50) -> ("StringsAndValues[]"=w56:T2)  [unwired: 1 in, 2 out]
      n6 = for {
        tunnel: w56 -> [w63] mode=indexing
        tunnel: [w60] -> w55 mode=indexing
        n7 = Unbundle(w63) -> ("String"=w61:string, "Value"=w62:i32)
        n8 = Bundle("Value"=w62, "String"=w61) -> (w60:cluster{"Value":i32, "String":string})  [unwired: 1 in]
      }
      n9 = Sort 1D Array(array=w55) -> (sorted array=w54:cluster{"Value":i32, "String":string}[])
      n10 = for {
        tunnel: w54 -> [w59] mode=indexing
        tunnel: [w57] -> w53 mode=indexing
        tunnel: [w58] -> w52 mode=indexing
        n11 = Unbundle(w59) -> ("Value"=w57:i32, "String"=w58:string)
      }
    }
  }
  n12 = call <vilib>:"Application Directory.vi"() -> ("Application Directory"=w43:path)
  n13 = Temporary Directory() -> (w46:path)
  n14 = Build Path(base path=w43, name or relative path=path "Temp") -> (appended path=w11:path)
  n15 = Format Into String(format string="%s", "Type") -> (resulting string=w21:string)  [unwired: 2 in, 1 out]
  n16 = for {
    N: 100 -> [_]
    tunnel: [w68] -> w44
    tunnel: w46 -> [w69]
    tunnel: [w67] -> w29
    stop <- w67 continue-if-true
    n17 = Random Number (0-1)() -> (number: 0 to 1=w72:dbl)
    n18 = Multiply(x=w72, y=1000000.0) -> (x*y=w66:dbl)
    n19 = Format Into String(format string="lvtemp%d", w66) -> (resulting string=w65:string)  [unwired: 2 in, 1 out]
    n20 = Build Path(base path=w69, name or relative path=w65) -> (appended path=w70:path)
    n21 = Create Folder(path (use dialog)=w70) -> (created path=w68:path, error out=w67:errorcluster)  [unwired: 2 in, 1 out]
  }
  n22 = Build Path(base path=w11, name or relative path=w21) -> (appended path=w10:path)
  n23 = Empty String/Path?(string/path="OutputDir") -> (empty?=w14:bool)
  n24 = Not A Number/Path/Refnum?(number/path/refnum="OutputDir") -> (NaN/Path/Refnum?=w15:bool)
  n25 = Or(x=w14, y=w15) -> (x .or. y?=w13:bool)
  n26 = Select(t=w10, s=w13, f="OutputDir") -> (s? t:f=w9:path)
  n27 = Create Folder(path (use dialog)=w9, error in="error in (no error)") -> (error out=w41:errorcluster)  [unwired: 1 in, 2 out]
  n28 = for {
    tunnel: w6 -> [w81] mode=indexing
    tunnel: w5 -> [w73] mode=indexing
    shift-right: [w79] -> w17
    shift-left: "" -> [w78]
    w76 = TRUE ("replace all? (F)")
    n29 = call <vilib>:"Space Constant.vi"() -> ("String"=w77:string)
    n30 = Search and Replace String(replace all?=w76, multiline?=w76, input string=w73, search string="[\\r\\n]+", replace string=w77) -> (result string=w74:string)  [unwired: 3 in, 3 out]
    n31 = Format Into String(format string="%d=%s\n", initial string=w78, w81, w74) -> (resulting string=w79:string)  [unwired: 1 in, 1 out]
  }
  n32 = call <vilib>:"Clear Errors.vi"("error in (no error)"=w41, "specific error code to clear (0: all)"=10) -> ("error out"=w32:errorcluster)  [unwired: 4 in, 1 out]
  n33 = Merge Errors(w29, w32) -> (w30:errorcluster)
  n34 = Format Into String(format string="_%s.txt", w21) -> (resulting string=w34:string)  [unwired: 2 in, 1 out]
  n35 = Build Path(base path=w9, name or relative path=w34) -> (appended path=w38:path)
  n36 = Build Path(base path=w9, name or relative path="_Scripting.txt" ("format string")) -> (appended path=w19:path)
  n37 = Write to Text File(file (use dialog)=w19, text=w17, error in=w30) -> (refnum out=w22:refnum<file>, error out=w24:errorcluster)  [unwired: 1 in, 1 out]
  n38 = Close File(refnum=w22, error in=w24) -> (error out=w23:errorcluster)  [unwired: 1 out]
  n39 = Unbundle By Name("Skip") -> ("Functions"=w1:i32[], "Controls"=w2:i32[])
  n40 = Open/Create/Replace File(file path (use dialog)=w38, error in=w23, operation (0:open)=T1."replace or create") -> (refnum out=w36:refnum<file>, error out=w31:errorcluster)  [unwired: 3 in, 1 out]
  n41 = while {
    tunnel: w44 -> [w92]
    shift-right: [w99] -> w47
    shift-left: w31 -> [w100]
    shift-right: [w91] -> _
    shift-left: 0 -> [w98]
    shift-right: [w93] -> w27
    shift-left: w36 -> [w94]
    tunnel: w9 -> [w95]
    tunnel: [w86] -> w26
    tunnel: [w90] -> w16 mode=indexing if=w89
    tunnel: w6 -> [w88]
    tunnel: w5 -> [w87]
    tunnel: "Type" -> [w85]
    tunnel: w2 -> [w84]
    tunnel: w1 -> [w83]
    stop <- w96 stop-if-true
    w82 = i16 32767  # Max ID
    # "next id"
    n42 = New VI(8:w100) -> (0:w101:errorcluster, 3:w105:refnum<vi>)  [unwired: 6 in]
    n43 = invoke class="VI" method="FP.Open"(reference=w105, error in=w101) -> (reference out=w103:refnum<vi>, error out=w102:errorcluster)  [unwired: 3 in, 3 out]
    n44 = property class="VI"(reference=w103, error in=w102, "BDWin.Open"=TRUE ("Block Diagram Window:Open")) -> (reference out=w107:refnum<vi>, error out=w106:errorcluster)
    n45 = case shown="\"Controls\"" w85 {
      tunnel: w107 -> [w130 w321]
      tunnel: w106 -> [w129 w320]
      tunnel: w98 -> [w127 w318]
      tunnel: [w122 w313] -> w97
      tunnel: [w121 w312] -> w96
      tunnel: w95 -> [w120 w311]
      tunnel: w94 -> [w117 w309]
      tunnel: [w116 w308] -> w93
      tunnel: w92 -> [w110 w302]
      tunnel: [w115 w307] -> w90
      tunnel: [w114 w306] -> w89
      tunnel: w88 -> [w113 w305]
      tunnel: w87 -> [w112 w304]
      tunnel: [w110 w302] -> w86
      tunnel: w84 -> [_ w300]
      tunnel: w83 -> [w109 _]
      tunnel: w82 -> [w108 w299]
      frame "Functions" {
        n46 = property class="VI"(reference=w130, error in=w129) -> (reference out=w124:refnum<vi>, error out=w128:errorcluster, "Diagram"=w118:refnum<vi>)
        n47 = To Long Integer(number=w108) -> (32bit integer=w119:i32)
        n48 = while {
          tunnel: w118 -> [w148]
          shift-right: [w136] -> w126
          shift-left: w128 -> [w149]
          shift-right: [w138] -> w125
          shift-left: w127 -> [w134]
          tunnel: w109 -> [w146]
          tunnel: [w142] -> w123
          tunnel: w119 -> [w139]
          tunnel: [w140] -> w121
          tunnel: w113 -> [w133]
          tunnel: w112 -> [w132]
          tunnel: [w131] -> w111
          stop <- w141 stop-if-true
          n49 = Equal?(x=w146, y=w134) -> (x = y?=w147:bool[])
          n50 = Search 1D Array(1D array=w133, element=w134) -> (index of element=w135:i32)  [unwired: 1 in]
          n51 = Or Array Elements(Boolean array=w147) -> (logical OR=w145:bool)
          n52 = case shown="False" w145 {
            tunnel: w149 -> [w158 w163]
            tunnel: w148 -> [w157 _]
            tunnel: [w154 w163] -> w143
            tunnel: [w153 _] -> w142
            tunnel: w134 -> [w152 _]
            frame False {
              w150 = refnum<vi> refnum  # Generic
              n53 = New VI Object(vi object class=w150, owner refnum=w157, style=w152, position/next to=T3 {"Horizontal"=0, "Vertical"=0} ("location"), 8:w158) -> (object refnum=w156:refnum<vi>, 0:w155:errorcluster)  [unwired: 3 in]
              n54 = case shown="No Error" w155 {
                selector: w155 -> [w161 _]
                tunnel: w156 -> [w159 w162]
                tunnel: [w161 _] -> w154
                tunnel: [TRUE _] -> w153
                frame No Error {
                  n55 = Close Reference(reference=w159) -> ()  [unwired: 1 in, 1 out]
                }
                frame Error {
                  n56 = invoke class="Gen" method="Delete"(reference=w162) -> ()  [unwired: 2 in, 3 out]
                }
              }
            }
            frame True {
            }
          }
          n57 = Index Array(array=w132, index=w135) -> (element=w131:string)
          "Name" <- w131
          n58 = Increment(x=w134) -> (x+1=w144:i32)
          n59 = call <vilib>:"Clear Errors.vi"("error in (no error)"=w143) -> ("error out"=w136:errorcluster)  [unwired: 5 in, 1 out]
          n60 = Select(t=w134, s=w142, f=w144) -> (s? t:f=w138:i32)
          n61 = Greater Or Equal?(x=w138, y=w139) -> (x >= y?=w140:bool)
          n62 = Subtract(x=w139, y=w138) -> (x-y=→"Remaining":i32)
          n63 = Or(x=w142, y=w140) -> (x .or. y?=w141:bool)
          "Current" <- w134
        }
        n64 = case shown="True" w123 {
          tunnel: w126 -> [w170 w177]
          tunnel: w125 -> [w164 w173]
          tunnel: w124 -> [w168 w179]
          tunnel: w110 -> [_ w181]
          tunnel: [w167 w180] -> w122
          tunnel: w120 -> [_ w178]
          tunnel: w118 -> [_ w176]
          tunnel: w117 -> [w165 w175]
          tunnel: [w165 w174] -> w116
          tunnel: [w164 w173] -> w115
          tunnel: [_ TRUE] -> w114
          tunnel: w111 -> [_ w171]
          frame False {
            n65 = invoke class="VI" method="FP.Close"(reference=w168, error in=w170) -> (reference out=w166:refnum<vi>, error out=w169:errorcluster)  [unwired: 1 in, 1 out]
            n66 = Close Reference(reference=w166, error in (no error)=w169) -> (error out=w167:errorcluster)
          }
          frame True {
            n67 = stacked-sequence {
              seq-local: [w182 _] -> [_ w266]
              tunnel: w173 -> [w184 w272]
              tunnel: w181 -> [_ w291]
              tunnel: [_ w286] -> w180
              tunnel: w179 -> [_ w283]
              tunnel: w178 -> [_ w271]
              tunnel: w177 -> [w202 w282]
              tunnel: w176 -> [w203 _]
              tunnel: w175 -> [w186 _]
              tunnel: [w185 _] -> w174
              tunnel: w171 -> [w183 _]
              frame #0 {
                n68 = property class="TopLvlDiag"(reference=w203, error in=w202) -> (reference out=w200:refnum<vi>, error out=w201:errorcluster, "Nodes[]"=w204:refnum<vi>[])
                n69 = stacked-sequence {
                  tunnel: w204 -> [w227 w236 w262]
                  tunnel: w201 -> [w225 w234 w261]
                  tunnel: w200 -> [_ _ _]
                  tunnel: w184 -> [w222 _ _]
                  tunnel: w183 -> [w216 _ _]
                  tunnel: [w222 _ _] -> w198
                  tunnel: [w211 _ _] -> w197
                  tunnel: [w217 _ _] -> w196
                  tunnel: [w221 _ _] -> w195
                  tunnel: [w206 _ _] -> w194
                  tunnel: [w205 _ _] -> w193
                  tunnel: [_ w229 _] -> w188
                  tunnel: [_ w228 _] -> w187
                  frame #0 {
                    w209 = TRUE ("replace all? (F)")
                    w214 = TRUE ("replace all? (F)")
                    w219 = TRUE ("replace all? (F)")
                    n70 = Index Array(array=w227) -> (element=w226:refnum<vi>)  [unwired: 1 in]
                    n71 = property class="Node"(reference=w226, error in=w225) -> (reference out=w223:refnum<vi>, error out=w224:errorcluster, "ClassID"=w221:u32, "ClassName"=w207:string, "MasterRect"=w205:T4)
                    n72 = property class="Node"(reference=w223, error in=w224) -> ("Label.Text"=w212:string)  [unwired: 2 out]
                    n73 = call <vilib>:"Space Constant.vi"() -> ("String"=w218:string)
                    n74 = call <vilib>:"Space Constant.vi"() -> ("String"=w215:string)
                    n75 = call <vilib>:"Space Constant.vi"() -> ("String"=w208:string)
                    n76 = Search and Replace String(replace all?=w219, multiline?=w219, input string=w216, search string="[\\r\\n]+", replace string=w218) -> (result string=w217:string)  [unwired: 3 in, 3 out]
                    n77 = Search and Replace String(replace all?=w214, multiline?=w214, input string=w212, search string="[\\r\\n]+", replace string=w215) -> (result string=w211:string)  [unwired: 3 in, 3 out]
                    n78 = Search and Replace String(replace all?=w209, multiline?=w209, input string=w207, search string="[\\r\\n]+", replace string=w208) -> (result string=w206:string)  [unwired: 3 in, 3 out]
                  }
                  frame #1 {
                    n79 = Index Array(array=w236) -> (element=w235:refnum<vi>)  [unwired: 1 in]
                    n80 = property class="Node"(reference=w235, error in=w234) -> (error out=w233:errorcluster, "Terms[]"=w232:refnum<vi>[])  [unwired: 1 out]
                    n81 = Array Size(array=w232) -> (size(s)=w229:i32)
                    n82 = for {
                      tunnel: w233 -> [w244]
                      tunnel: w232 -> [w243] mode=indexing
                      shift-right: [w241] -> w228
                      shift-left: "" -> [w240]
                      tunnel: "term/%d=%d,%d,%d,%d,%s,#%06x,%s\n" ("format string") -> [w237]
                      i -> [w242]
                      w246 = TRUE ("replace all? (F)")
                      n83 = property class="Term"(reference=w243, error in=w244) -> (reference out=w238:refnum<vi>, error out=w239:errorcluster, "MasterRect"=w253:T4, "IsSource"=w252:bool, "Name"=w251:string, "Data Type"=w250:variant)
                      n84 = Close Reference(reference=w238, error in (no error)=w239) -> ()  [unwired: 1 out]
                      n85 = invoke class="App" method="Data Type Color"("Data Type"=w250) -> ("Data Type Color"=w249:u32)  [unwired: 3 in, 3 out]
                      n86 = call <vilib>:"Space Constant.vi"() -> ("String"=w256:string)
                      n87 = Select(t="o", s=w252, f="i") -> (s? t:f=w255:string)
                      n88 = Search and Replace String(replace all?=w246, multiline?=w246, input string=w251, search string="[\\r\\n]+", replace string=w256) -> (result string=w254:string)  [unwired: 3 in, 3 out]
                      n89 = Unbundle(w253) -> ("Left"=w260:i16, "Top"=w259:i16, "Right"=w258:i16, "Bottom"=w257:i16)
                      n90 = Format Into String(format string=w237, initial string=w240, w242, w260, w259, w258, w257, w255, w249, w254) -> (resulting string=w241:string)  [unwired: 1 in, 1 out]
                    }
                  }
                  frame #2 {
                    n91 = Close Reference(reference=w262, error in (no error)=w261) -> ()  [unwired: 1 out]
                  }
                }
                n92 = Unbundle(w193) -> ("Left"=w192:i16, "Top"=w191:i16, "Right"=w190:i16, "Bottom"=w189:i16)
                n93 = Format Into String(format string="[%d]\nname=%s\nring=%s\nclass=%d,%s\nrect=%d,%d,%d,%d\nterms=%d\n%s\n", w198, w197, w196, w195, w194, w192, w191, w190, w189, w188, w187) -> (resulting string=w182:string)  [unwired: 2 in, 1 out]
                "Info" <- w182
                n94 = Write to Text File(file (use dialog)=w186, text=w182) -> (refnum out=w185:refnum<file>)  [unwired: 2 in, 2 out]
              }
              frame #1 {
                n95 = invoke class="VI" method="BD.Get Image Scaled"(reference=w283, error in=w282, "img depth"=24 ("Image Depth")) -> (reference out=w281:refnum<vi>, error out=w279:errorcluster, "img data"=w265:T5)  [unwired: 4 in, 4 out]
                n96 = invoke class="VI" method="VI Icon.Set from Image Data"(reference=w281, error in=w279, "ImageData"=w265) -> (reference out=w280:refnum<vi>, error out=w278:errorcluster)  [unwired: 3 in, 4 out]
                n97 = Format Into String(format string="%d.txt", w272) -> (resulting string=w273:string)  [unwired: 2 in, 1 out]
                n98 = Format Into String(format string="%d.png", w272) -> (resulting string=w293:string)  [unwired: 2 in, 1 out]
                n99 = Format Into String(format string="%d.vi", w272) -> (resulting string=w297:string)  [unwired: 2 in, 1 out]
                n100 = Build Path(base path=w271, name or relative path=w273) -> (appended path=w270:path)
                n101 = Build Path(base path=w271, name or relative path=w293) -> (appended path=w264:path)
                "Last Snippet (.png)" <- w264
                n102 = Build Path(base path=w291, name or relative path=w297) -> (appended path=w285:path)
                n103 = Select(t=w279, s=w278, f=w278) -> (s? t:f=w277:errorcluster)
                n104 = invoke class="VI" method="Save.Instrument"(reference=w280, error in=w277, "Path to saved file"=w285) -> (reference out=w289:refnum<vi>, error out=w294:errorcluster)  [unwired: 3 in, 4 out]
                n105 = call <vilib>:"Clear Errors.vi"("error in (no error)"=w294) -> ("error out"=w276:errorcluster)  [unwired: 5 in, 1 out]
                n106 = invoke class="VI" method="FP.Close"(reference=w289, error in=w276) -> (reference out=w287:refnum<vi>, error out=w290:errorcluster)  [unwired: 1 in, 1 out]
                n107 = Close Reference(reference=w287, error in (no error)=w290) -> (error out=w288:errorcluster)
                n108 = call "Write VI Snippet.vi"("error in (no error)"=w288, "Image Data"=w265, "VI Path (.vi)"=w285, "VI Snippet (.png)"=w264) -> ("error out"=w295:errorcluster)  [unwired: 7 in]
                n109 = call <vilib>:"Draw Flattened Pixmap.vi"("image data"=w265) -> ("new picture"=→"Image":picture)  [unwired: 8 in]
                n110 = call <vilib>:"Clear Errors.vi"("error in (no error)"=w295) -> ("error out"=w284:errorcluster)  [unwired: 5 in, 1 out]
                n111 = Write to Text File(file (use dialog)=w270, text=w266, error in=w284) -> (refnum out=w268:refnum<file>, error out=w275:errorcluster)  [unwired: 1 in, 1 out]
                n112 = Close File(refnum=w268, error in=w275) -> (error out=w269:errorcluster)  [unwired: 1 out]
                n113 = call <vilib>:"Clear Errors.vi"("error in (no error)"=w269) -> ("error out"=w267:errorcluster)  [unwired: 5 in, 1 out]
                n114 = Delete(path (use dialog)=w285, error in=w267) -> (error out=w286:errorcluster)  [unwired: 3 in, 2 out]
              }
            }
            "Last" <- w173
          }
        }
      }
      frame "Controls" {
        n115 = property class="VI"(reference=w321, error in=w320) -> (reference out=w315:refnum<vi>, error out=w319:errorcluster, "Panel"=w301:refnum<vi>)
        n116 = To Long Integer(number=w299) -> (32bit integer=w310:i32)
        n117 = while {
          tunnel: w301 -> [w339]
          shift-right: [w328] -> w317
          shift-left: w319 -> [w340]
          shift-right: [w329] -> w316
          shift-left: w318 -> [w322]
          tunnel: w300 -> [w337]
          tunnel: [w333] -> w314
          tunnel: w310 -> [w330]
          tunnel: [w331] -> w312
          tunnel: w305 -> [w326]
          tunnel: w304 -> [w325]
          tunnel: [w324] -> w303
          stop <- w332 stop-if-true
          n118 = Equal?(x=w337, y=w322) -> (x = y?=w338:bool[])
          n119 = Search 1D Array(1D array=w326, element=w322) -> (index of element=w327:i32)  [unwired: 1 in]
          n120 = Or Array Elements(Boolean array=w338) -> (logical OR=w336:bool)
          n121 = local write "Current"(w322) -> ()
          n122 = case shown="False" w336 {
            tunnel: w340 -> [w349 w354]
            tunnel: w339 -> [w348 _]
            tunnel: [w345 w354] -> w334
            tunnel: [w344 _] -> w333
            tunnel: w322 -> [w343 _]
            frame False {
              w341 = refnum<vi> refnum  # Generic
              n123 = New VI Object(vi object class=w341, owner refnum=w348, style=w343, position/next to=T3 {"Horizontal"=0, "Vertical"=0} ("location"), 8:w349) -> (object refnum=w347:refnum<vi>, 0:w346:errorcluster)  [unwired: 3 in]
              n124 = case shown="No Error" w346 {
                selector: w346 -> [w352 _]
                tunnel: w347 -> [w350 w353]
                tunnel: [w352 _] -> w345
                tunnel: [TRUE _] -> w344
                frame No Error {
                  n125 = Close Reference(reference=w350) -> ()  [unwired: 1 in, 1 out]
                }
                frame Error {
                  n126 = invoke class="Gen" method="Delete"(reference=w353) -> ()  [unwired: 2 in, 3 out]
                }
              }
            }
            frame True {
            }
          }
          n127 = Index Array(array=w325, index=w327) -> (element=w324:string)
          n128 = Increment(x=w322) -> (x+1=w335:i32)
          n129 = call <vilib>:"Clear Errors.vi"("error in (no error)"=w334) -> ("error out"=w328:errorcluster)  [unwired: 5 in, 1 out]
          n130 = Select(t=w322, s=w333, f=w335) -> (s? t:f=w329:i32)
          n131 = Greater Or Equal?(x=w329, y=w330) -> (x >= y?=w331:bool)
          n132 = Subtract(x=w330, y=w329) -> (x-y=w323:i32)
          n133 = Or(x=w333, y=w331) -> (x .or. y?=w332:bool)
          n134 = local write "Remaining"(w323) -> ()
          n135 = local write "Name"(w324) -> ()
        }
        n136 = case shown="True" w314 {
          tunnel: w317 -> [w361 w368]
          tunnel: w316 -> [w355 w362]
          tunnel: w315 -> [w359 w370]
          tunnel: w302 -> [_ w372]
          tunnel: [w358 w371] -> w313
          tunnel: w311 -> [_ w369]
          tunnel: w301 -> [_ w367]
          tunnel: w309 -> [w356 w366]
          tunnel: [w356 w365] -> w308
          tunnel: [w355 w362] -> w307
          tunnel: [_ TRUE] -> w306
          tunnel: w303 -> [_ w363]
          frame False {
            n137 = invoke class="VI" method="FP.Close"(reference=w359, error in=w361) -> (reference out=w357:refnum<vi>, error out=w360:errorcluster)  [unwired: 1 in, 1 out]
            n138 = Close Reference(reference=w357, error in (no error)=w360) -> (error out=w358:errorcluster)
          }
          frame True {
            n139 = stacked-sequence {
              seq-local: [w374 _] -> [_ w465]
              tunnel: w362 -> [w376 w471]
              tunnel: w372 -> [_ w489]
              tunnel: [_ w484] -> w371
              tunnel: w370 -> [_ w461]
              tunnel: w369 -> [_ w470]
              tunnel: w368 -> [w394 w481]
              tunnel: w367 -> [w395 _]
              tunnel: w366 -> [w378 _]
              tunnel: [w377 _] -> w365
              tunnel: w363 -> [w375 _]
              frame #0 {
                n140 = property class="Pnl"(reference=w395, error in=w394) -> (reference out=w392:refnum<vi>, error out=w393:errorcluster, "Controls[]"=w396:refnum<vi>[], "AllObjs[]"=w373:refnum<vi>[])
                n141 = stacked-sequence {
                  tunnel: w396 -> [w401 w425 w456]
                  tunnel: w393 -> [w421 w426 w455]
                  tunnel: w392 -> [_ _ _]
                  tunnel: w376 -> [w420 _ _]
                  tunnel: w375 -> [w414 _ _]
                  tunnel: [w420 _ _] -> w390
                  tunnel: [w409 _ _] -> w389
                  tunnel: [w415 _ _] -> w388
                  tunnel: [w419 _ _] -> w387
                  tunnel: [w404 _ _] -> w386
                  tunnel: [w403 _ _] -> w385
                  tunnel: [_ w422 _] -> w380
                  tunnel: [_ w427 _] -> w379
                  tunnel: w373 -> [w402 _ w454]
                  frame #0 {
                    w407 = TRUE ("replace all? (F)")
                    w412 = TRUE ("replace all? (F)")
                    w417 = TRUE ("replace all? (F)")
                    n142 = Index Array(array=w401) -> (element=w397:refnum<vi>)  [unwired: 1 in]
                    n143 = Index Array(array=w402) -> (element=w399:refnum<vi>)  [unwired: 1 in]
                    n144 = Not A Number/Path/Refnum?(number/path/refnum=w397) -> (NaN/Path/Refnum?=w400:bool)
                    n145 = Select(t=w399, s=w400, f=w397) -> (s? t:f=w398:refnum<vi>)
                    n146 = property class="GObj"(reference=w398, error in=w421) -> ("ClassID"=w419:u32, "ClassName"=w405:string, "MasterRect"=w403:T4)  [unwired: 2 out]
                    n147 = property class="Ctl"(reference=w397) -> ("Label.Text"=w410:string)  [unwired: 1 in, 2 out]
                    n148 = call <vilib>:"Space Constant.vi"() -> ("String"=w416:string)
                    n149 = call <vilib>:"Space Constant.vi"() -> ("String"=w413:string)
                    n150 = call <vilib>:"Space Constant.vi"() -> ("String"=w406:string)
                    n151 = Search and Replace String(replace all?=w417, multiline?=w417, input string=w414, search string="[\\r\\n]+", replace string=w416) -> (result string=w415:string)  [unwired: 3 in, 3 out]
                    n152 = Search and Replace String(replace all?=w412, multiline?=w412, input string=w410, search string="[\\r\\n]+", replace string=w413) -> (result string=w409:string)  [unwired: 3 in, 3 out]
                    n153 = Search and Replace String(replace all?=w407, multiline?=w407, input string=w405, search string="[\\r\\n]+", replace string=w406) -> (result string=w404:string)  [unwired: 3 in, 3 out]
                  }
                  frame #1 {
                    n154 = for {
                      tunnel: w426 -> [w438]
                      tunnel: w425 -> [w431] mode=indexing
                      tunnel: "term/%d=%d,%d,%d,%d,%s,#%06x,%s\n" ("format string") -> [w430]
                      shift-right: [w453] -> w427
                      shift-left: "" -> [w429]
                      w440 = TRUE ("replace all? (F)")
                      n155 = property class="Ctl"(reference=w431, error in=w438) -> (reference out=w437:refnum<vi>, error out=w428:errorcluster, "MasterRect"=w445:T4, "Indicator"=w444:bool)
                      n156 = property class="Ctl"(reference=w437, error in=w428) -> (reference out=w435:refnum<vi>, "Label.Text"=w436:string)  [unwired: 1 out]
                      n157 = property class="Ctl"(reference=w435, error in=w428) -> (reference out=w434:refnum<vi>, "Value"=w433:variant)  [unwired: 1 out]
                      n158 = Close Reference(reference=w434) -> ()  [unwired: 1 in, 1 out]
                      n159 = invoke class="App" method="Data Type Color"("Data Type"=w433) -> ("Data Type Color"=w443:u32)  [unwired: 3 in, 3 out]
                      n160 = call <vilib>:"Space Constant.vi"() -> ("String"=w448:string)
                      n161 = Select(t="i" ("f"), s=w444, f="o") -> (s? t:f=w447:string)
                      n162 = Search and Replace String(replace all?=w440, multiline?=w440, input string=w436, search string="[\\r\\n]+", replace string=w448) -> (result string=w446:string)  [unwired: 3 in, 3 out]
                      n163 = Unbundle(w445) -> ("Left"=w452:i16, "Top"=w451:i16, "Right"=w450:i16, "Bottom"=w449:i16)
                      n164 = Format Into String(format string=w430, initial string=w429, 0 ("input 1"), w452, w451, w450, w449, w447, w443, w446) -> (resulting string=w453:string)  [unwired: 1 in, 1 out]
                    }
                    n165 = Array Size(array=w425) -> (size(s)=w422:i32)
                  }
                  frame #2 {
                    n166 = Close Reference(reference=w456, error in (no error)=w455) -> ()  [unwired: 1 out]
                    n167 = Close Reference(reference=w454) -> ()  [unwired: 1 in, 1 out]
                  }
                }
                n168 = Unbundle(w385) -> ("Left"=w384:i16, "Top"=w383:i16, "Right"=w382:i16, "Bottom"=w381:i16)
                n169 = Format Into String(format string="[%d]\nname=%s\nring=%s\nclass=%d,%s\nrect=%d,%d,%d,%d\nterms=%d\n%s\n", w390, w389, w388, w387, w386, w384, w383, w382, w381, w380, w379) -> (resulting string=w374:string)  [unwired: 2 in, 1 out]
                n170 = Write to Text File(file (use dialog)=w378, text=w374) -> (refnum out=w377:refnum<file>)  [unwired: 2 in, 2 out]
                n171 = local write "Info"(w374) -> ()
              }
              frame #1 {
                n172 = invoke class="VI" method="BD.Get Image Scaled"(reference=w461, "img depth"=24 ("Image Depth")) -> ("img data"=w459:T5)  [unwired: 5 in, 6 out]
                n173 = invoke class="VI" method="FP.Get Image"(reference=w461, error in=w481, "visible area only"=FALSE ("Visible Area Only"), "image depth"=24 ("Image Depth")) -> (reference out=w480:refnum<vi>, error out=w478:errorcluster, "image data"=w462:T5)  [unwired: 2 in, 3 out]
                n174 = invoke class="VI" method="VI Icon.Set from Image Data"(reference=w480, error in=w478, "ImageData"=w459) -> (reference out=w479:refnum<vi>, error out=w477:errorcluster)  [unwired: 3 in, 4 out]
                n175 = Format Into String(format string="%d.txt", w471) -> (resulting string=w472:string)  [unwired: 2 in, 1 out]
                n176 = Format Into String(format string="%d.png", w471) -> (resulting string=w491:string)  [unwired: 2 in, 1 out]
                n177 = Format Into String(format string="%d.vi", w471) -> (resulting string=w494:string)  [unwired: 2 in, 1 out]
                n178 = Build Path(base path=w470, name or relative path=w472) -> (appended path=w469:path)
                n179 = Build Path(base path=w470, name or relative path=w491) -> (appended path=w457:path)
                n180 = Build Path(base path=w489, name or relative path=w494) -> (appended path=w483:path)
                n181 = Select(t=w478, s=w477, f=w477) -> (s? t:f=w476:errorcluster)
                n182 = invoke class="VI" method="Save.Instrument"(reference=w479, error in=w476, "Path to saved file"=w483) -> (reference out=w487:refnum<vi>, error out=w492:errorcluster)  [unwired: 3 in, 4 out]
                n183 = call <vilib>:"Clear Errors.vi"("error in (no error)"=w492) -> ("error out"=w475:errorcluster)  [unwired: 5 in, 1 out]
                n184 = invoke class="VI" method="FP.Close"(reference=w487, error in=w475) -> (reference out=w485:refnum<vi>, error out=w488:errorcluster)  [unwired: 1 in, 1 out]
                n185 = Close Reference(reference=w485, error in (no error)=w488) -> (error out=w486:errorcluster)
                n186 = call "Write VI Snippet.vi"("error in (no error)"=w486, "Image Data"=w462, "VI Path (.vi)"=w483, "VI Snippet (.png)"=w457) -> ("error out"=w493:errorcluster)  [unwired: 7 in]
                n187 = local write "Last Snippet (.png)"(w457) -> ()
                n188 = call <vilib>:"Draw Flattened Pixmap.vi"("image data"=w462) -> ("new picture"=w458:picture)  [unwired: 8 in]
                n189 = call <vilib>:"Clear Errors.vi"("error in (no error)"=w493) -> ("error out"=w482:errorcluster)  [unwired: 5 in, 1 out]
                n190 = local write "Image"(w458) -> ()
                n191 = Write to Text File(file (use dialog)=w469, text=w465, error in=w482) -> (refnum out=w467:refnum<file>, error out=w474:errorcluster)  [unwired: 1 in, 1 out]
                n192 = Close File(refnum=w467, error in=w474) -> (error out=w468:errorcluster)  [unwired: 1 out]
                n193 = call <vilib>:"Clear Errors.vi"("error in (no error)"=w468) -> ("error out"=w466:errorcluster)  [unwired: 5 in, 1 out]
                n194 = Delete(path (use dialog)=w483, error in=w466) -> (error out=w484:errorcluster)  [unwired: 3 in, 2 out]
              }
            }
            n195 = local write "Last"(w362) -> ()
          }
        }
      }
    }
    n196 = call <vilib>:"Clear Errors.vi"("error in (no error)"=w97) -> ("error out"=w99:errorcluster)  [unwired: 5 in, 1 out]
    n197 = Increment(x=w90) -> (x+1=w91:i32)
  }
  "error out" <- w47
  "IDs" <- w16
  n198 = Delete(path (use dialog)=w26, entire hierarchy (F)=TRUE) -> ()  [unwired: 3 in, 3 out]
  n199 = Close File(refnum=w27) -> ()  [unwired: 1 in, 2 out]
